vi "GetMembers.vi"(8 "error in (no error)":errorcluster, 11 "TecellaChannel in":refnum<class "TecellaChannel.lvclass">) -> (0 "error out":errorcluster, 1 "Channel":i8, 2 "TecellaClient.lvclass":refnum<class "TecellaClient.lvclass">, 3 "TecellaChannel out":refnum<class "TecellaChannel.lvclass">)   [LabVIEW 2009, in "TecellaChannel.lvclass"]
uses:
  TecellaChannel.lvclass
  TecellaClient/TecellaClient.lvclass
  TecellaChannel.lvclass/TecellaChannel.ctl
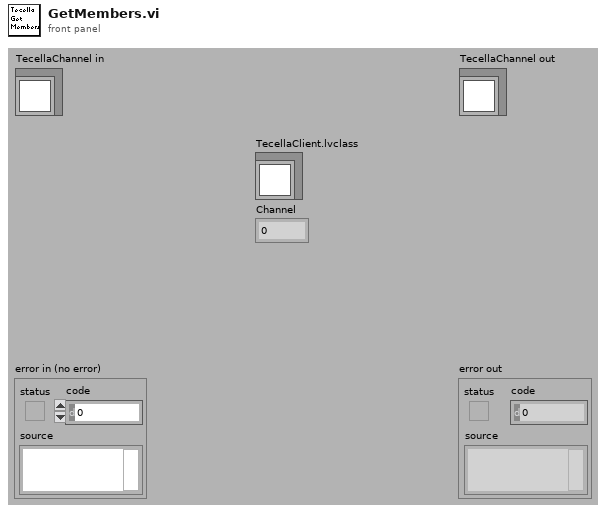
[diagram p1: front panel]
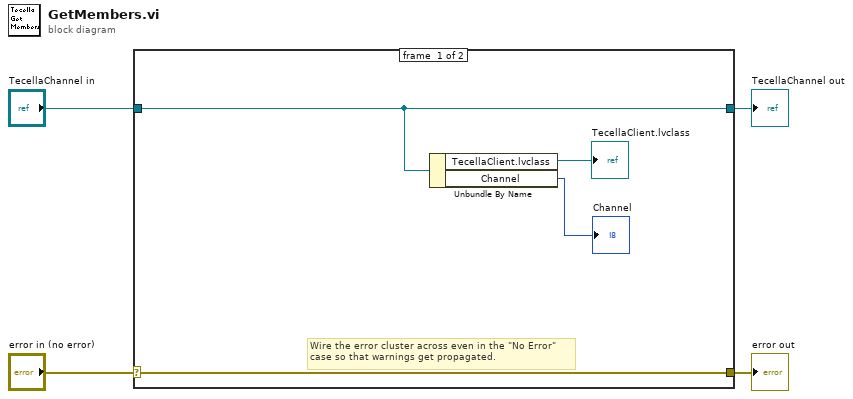
[diagram p0: block diagram]
diagram:
  n1 = case shown="No Error" "error in (no error)" {
    selector: "error in (no error)" -> [w8 w10]
    tunnel: [w8 w10] -> w3
    tunnel: [w7 w9] -> w1
    tunnel: "TecellaChannel in" -> [w7 w9]
    frame #0 {
      # "Wire the error cluster across even in the \"No Error\"\ncase so that warnings get propagated."
      n2 = Unbundle By Name(w7) -> ("TecellaClient.lvclass"=→"TecellaClient.lvclass":refnum<class "TecellaClient.lvclass">, "Channel"=→"Channel":i8)
    }
    frame #1 {
    }
  }
  "error out" <- w3
  "TecellaChannel out" <- w1
